vi "CFTS-Find Available Acoustic Systems.vi"(7 "Options":T1) -> (8 "Acoustic Systems":string[](array[string]))   [LabVIEW 2020]
uses:
  CFTS-Options.ctl
  fc558a3b-c7ad-4dad-962b-7f4d662fa22e.vi
  4d575e3f-91a0-470d-82b0-18b06768d028.vi
  <vilib>/Comparison/Less/Less Functor/Less Functor.lvclass
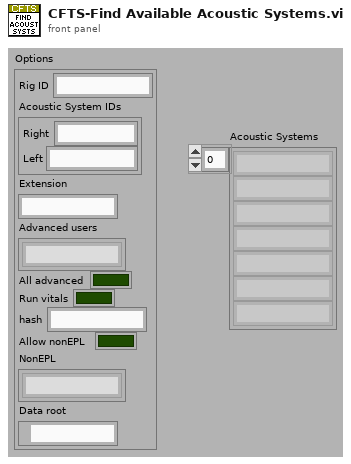
[diagram p1: front panel]
types:
  T1 = typedef "CFTS-Options.ctl" = cluster{"Rig ID":string, "Acoustic System IDs":cluster{"Right":string, "Left":string}, "Extension":string, "Advanced users":string[], "All advanced":bool, "Run vitals":bool, "hash":string, "Allow nonEPL":bool, "NonEPL":string[], "Data root":path}
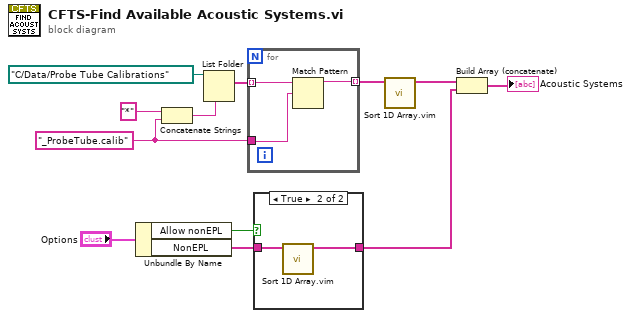
[diagram p0: block diagram]
diagram:
  w9 = "_ProbeTube.calib" ("string")
  n1 = Unbundle By Name("Options") -> ("Allow nonEPL"=w6:bool, "NonEPL"=w5:string[])
  n2 = Concatenate Strings("*" ("string"), w9) -> (w10:string)
  n3 = List Folder(path=path "C:/Data/Probe Tube Calibrations", pattern=w10) -> (filenames=w11:string[])  [unwired: 2 in, 3 out]
  n4 = for {
    tunnel: w11 -> [w15] mode=indexing
    tunnel: w9 -> [w14]
    tunnel: [w13] -> w4 mode=indexing
    n5 = Match Pattern(string=w15, regular expression=w14) -> (before substring=w13:string)  [unwired: 1 in, 3 out]
  }
  n6 = case shown="True" w6 {
    tunnel: w5 -> [_ w17]
    tunnel: [_ w16] -> w2
    frame False {
    }
    frame True {
      n7 = call "Sort 1D Array.vim"("unsorted array"=w17) -> ("sorted array"=w16:string[])  [unwired: 10 in]
    }
  }
  n8 = call "Sort 1D Array.vim"("unsorted array"=w4) -> ("sorted array"=w3:string[])  [unwired: 10 in]
  n9 = Build Array (concatenate)(w3, w2) -> (→"Acoustic Systems":string[])
